vi "Read Signal List.vi"(8 "error in":errorcluster, 11 "SLL in":refnum<class "SLL.lvclass">) -> (0 "error out":errorcluster, 3 "SLL out":refnum<class "SLL.lvclass">)   [LabVIEW 2023, in "SLL.lvlib" / "SLL.lvclass"]
uses:
  SLL.lvclass
  SLL.lvclass/SLL.ctl
  <vilib>/Utility/file.llb/Read Delimited Spreadsheet (string).vi
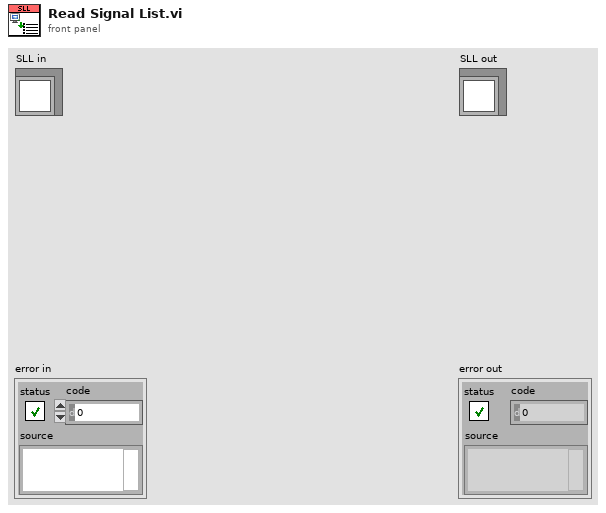
[diagram p1: front panel]
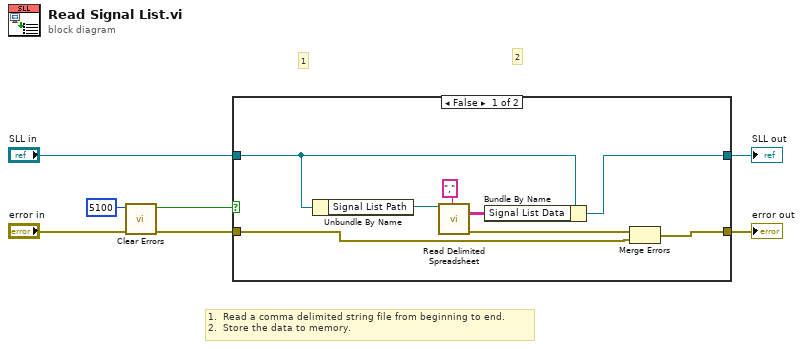
[diagram p0: block diagram]
diagram:
  # "1.  Read a comma delimited string file from beginning to end.\n2.  Store the data to memory."
  # "2"
  # "1"
  n1 = call <vilib>:"Clear Errors.vi"("error in (no error)"="error in", "specific error code to clear (0: all)"=5100) -> ("error out"=w1:errorcluster, "specific error cleared?"=w2:bool)  [unwired: 4 in]
  n2 = case shown="False" w2 {
    tunnel: [w9 w16] -> w7
    tunnel: [w12 w17] -> w5
    tunnel: "SLL in" -> [w15 w17]
    tunnel: w1 -> [w8 w16]
    frame False {
      n3 = Unbundle By Name(w15) -> ("Signal List Path"=w14:path)
      n4 = call-poly <vilib>:"Read Delimited Spreadsheet.vi"("file path (dialog if empty)"=w14, "delimiter (\\t)"="," ("delimiter (\\t)")) -> ("all rows"=w11:string[][], "error out"=w10:errorcluster)  [unwired: 8 in, 4 out]
      n5 = Bundle By Name(cluster=w15, "Signal List Data"=w11) -> (w12:refnum<class "SLL.lvclass">)
      n6 = Merge Errors(w10, w8) -> (w9:errorcluster)
    }
    frame True {
    }
  }
  "error out" <- w7
  "SLL out" <- w5
